vi "pathplan.vi"() -> ()   [LabVIEW 2016]
uses:
  <vilib>/imath/engines/lvmath2/RunTimeEngine/NodeEndStatement/NIMS_NodeEndStatement_Output.vi
  <instcachedir>/0/NIMS_NodeEndStatement_Output_53EC0D466D134D7ABD903AC30B43404B.lvgen/NIMS_NodeEndStatement_Output_53EC0D466D134D7ABD903AC30B43404B_011.vi
  <vilib>/imath/engines/lvmath2/RunTimeEngine/ErrorHandling/NIMS_Finalize Error.vi
panel:
  in  "串口设置（全场定位）":T1={"波特率"=115200, "数据位"=8, "校验"=enum."None", "停止位"=10, "流控制"=0} {"流控制" items=["无"=0, "XON/XOFF"=1, "RTS/CTS"=2, "DTR/DSR"=4]; "停止位" items=["1.0"=10, "1.5"=15, "2.0"=20]; "数据位" min=5 max=8 step=1; "波特率" items=["115200"=115200, "460800"=460800, "75"=75, "110"=110, "134"=134, "150"=150, "300"=300, "600"=600, "1200"=1200, "1800"=1800, "2400"=2400, "4800"=4800, "7200"=7200, "9600"=9600, "14400"=14400, "19200"=19200, "28800"=28800, "38400"=38400, "56000"=56000, "57600"=57600, "128000"=128000, "230400"=230400]}
  in  "全场定位串口":refnum<visa-resource-name>="ASRL4::INSTR" caption="全场定位模块"
  out "起点监视2":sgl[](array[numeric])
  in  "目标位置2":dbl[](array[numeric])=[6000.0, 1500.0]
  out "起点监视3":sgl[](array[numeric])
  in  "目标位置3":dbl[](array[numeric])=[2645.0, 2645.0]
  out "起点监视0":sgl[](array[numeric])
  in  "目标位置0":dbl[](array[numeric])=[12000.0, 0.0]
  in  "Key2(点3)":bool
  in  "Key1(点2)":bool
  in  "Key0(点1)":bool
  in  "speed_max":dbl=15000.0
  in  "发送写入":refnum<visa-resource-name>
  in  "车宽的一半":dbl=200.0
  out "起点监视1":sgl[](array[numeric])
  in  "目标位置1":dbl[](array[numeric])=[9355.0, 2645.0]
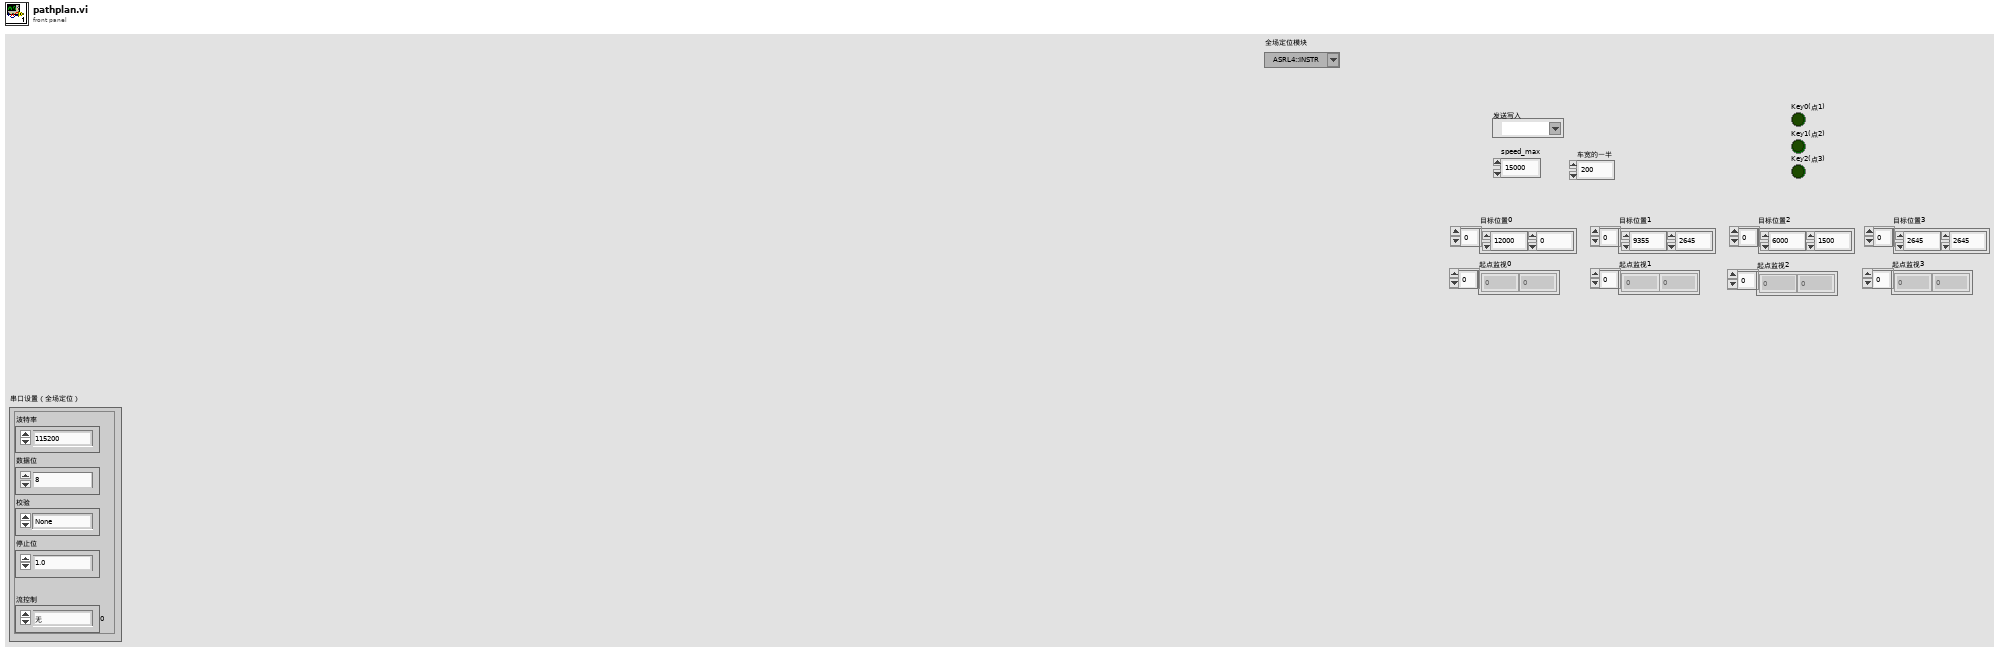
[diagram p1: front panel]
types:
  T1 = cluster{"波特率":u32, "数据位":u16, "校验":enum16{"None", "Odd", "Even", "Mark", "Space"}, "停止位":u16, "流控制":u16}
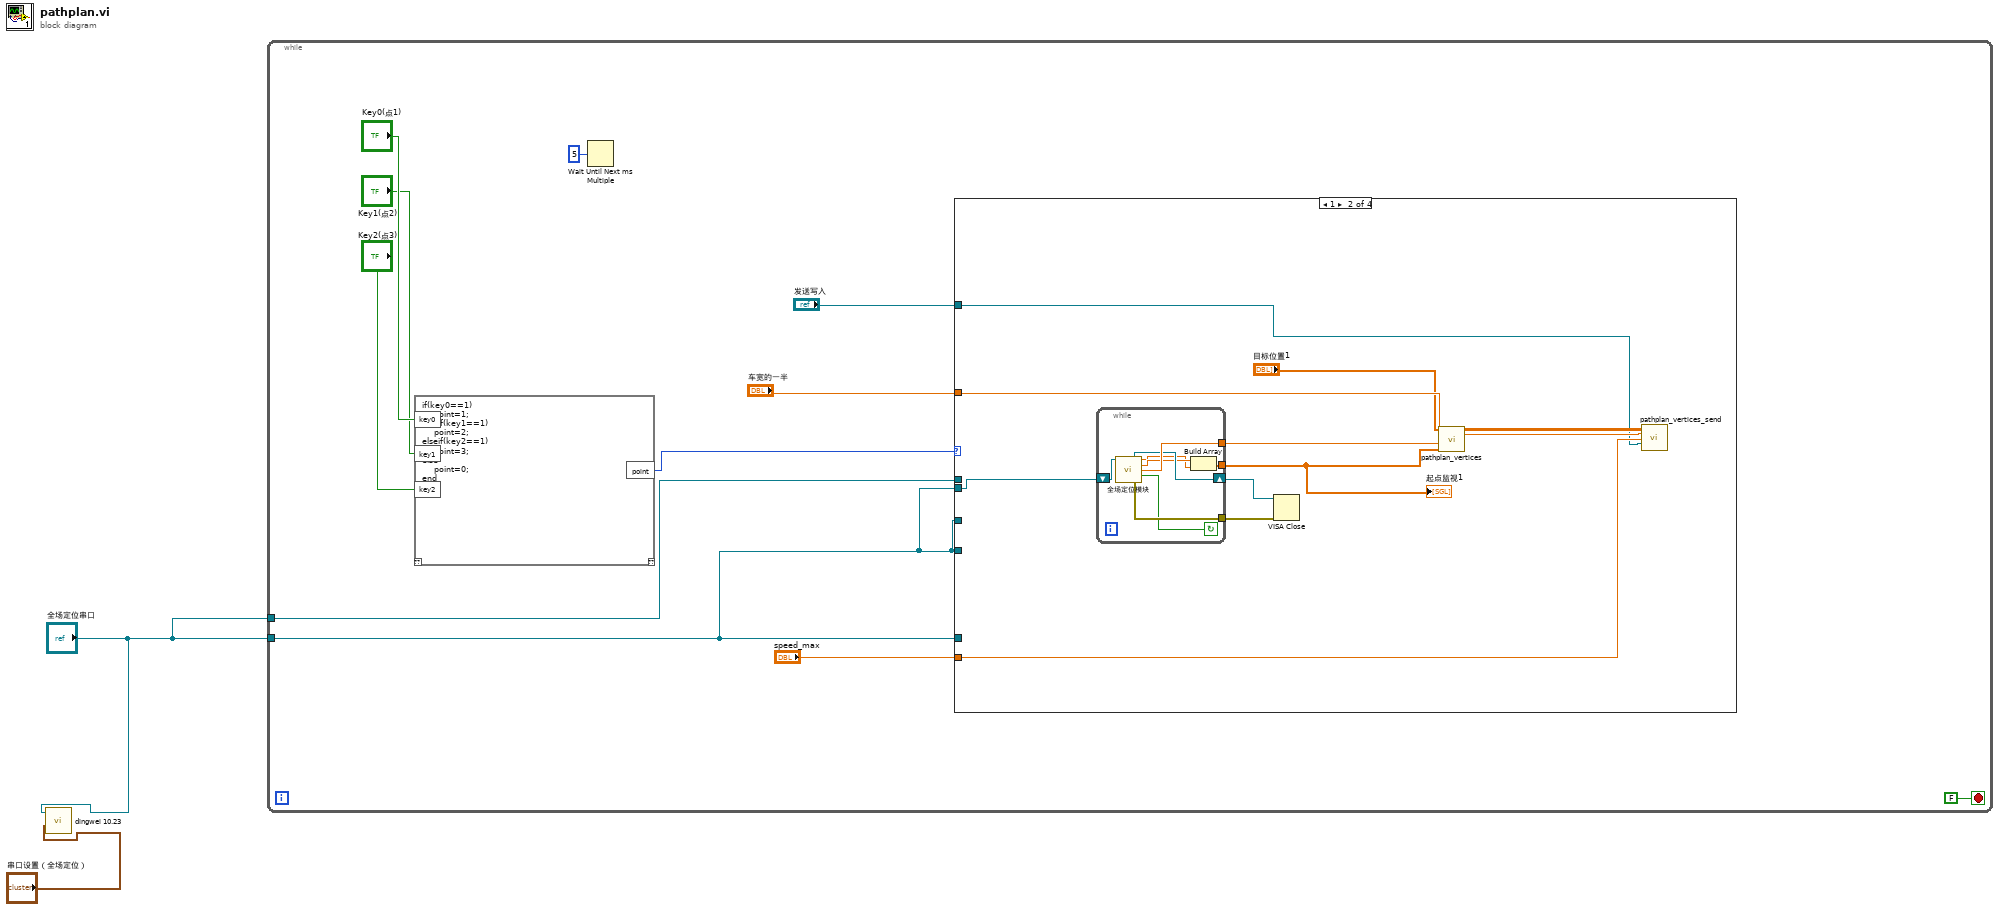
[diagram p0: block diagram]
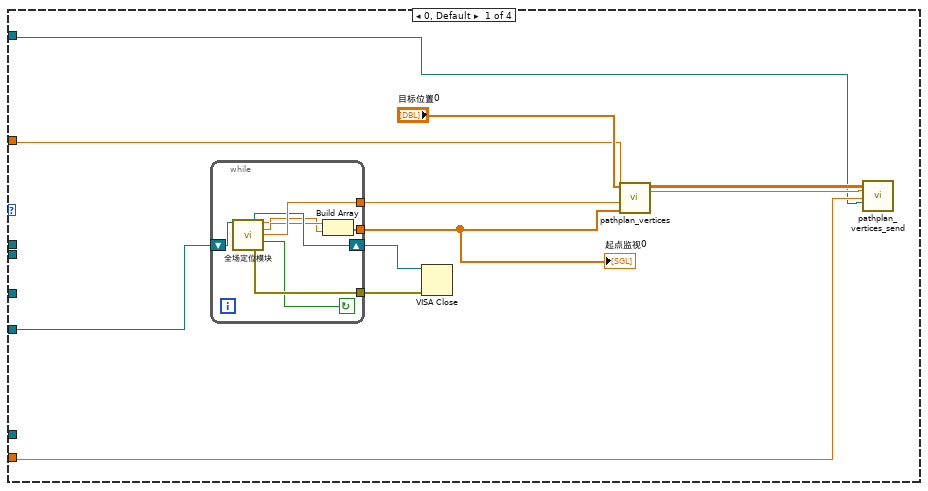
[diagram p2: hidden frame]
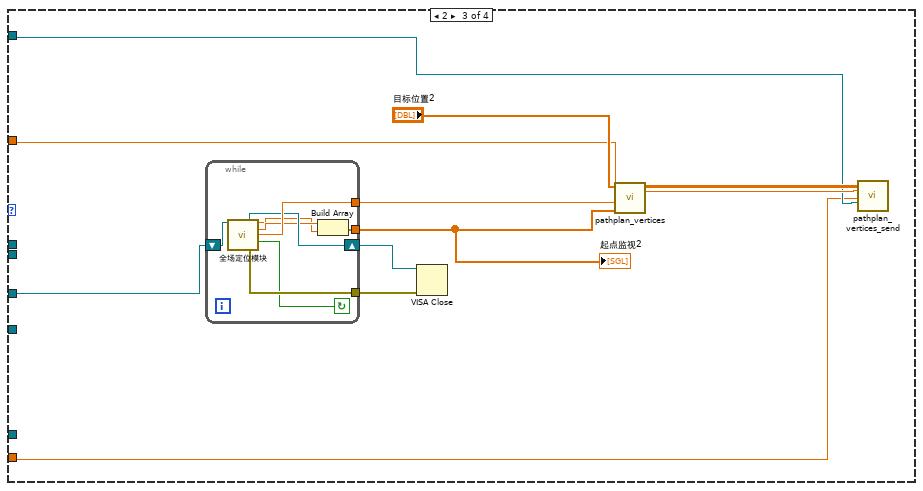
[diagram p3: hidden frame]
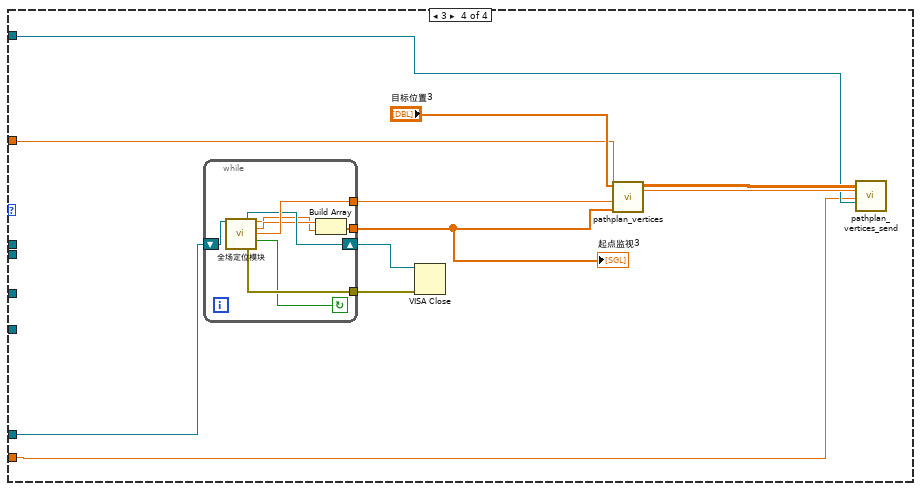
[diagram p4: hidden frame]
diagram:
  n1 = call "dingwei 10.23.vi"("串口设置（遥控器）"="串口设置（全场定位）", "VISA resource name"="全场定位串口") -> ()  [unwired: 10 in]
  n2 = while {
    tunnel: "全场定位串口" -> [w3]
    tunnel: "全场定位串口" -> [w4]
    stop <- FALSE stop-if-true
    n3 = mathscript code="if(key0==1)\n    point=1;\nelseif(key1==1)\n    point=2;\nelseif(key2==1)\n    point=3;\nelse\n    point=0;\nend"("key0"="Key0(点1)", "key1"="Key1(点2)", "key2"="Key2(点3)") -> ("point"=w7:i32)  [unwired: 1 in, 1 out]
    n4 = Wait Until Next ms Multiple(millisecond multiple=u32 5 ("等待时间（毫秒）")) -> ()  [unwired: 1 out]
    n5 = case shown="1" w7 {
      tunnel: "车宽的一半" -> [w92 w118 w130 w149]
      tunnel: "speed_max" -> [w93 w111 w129 w148]
      tunnel: "发送写入" -> [w91 w110 w131 w150]
      tunnel: w3 -> [_ _ _ w147]
      tunnel: w4 -> [_ _ _ _]
      tunnel: w3 -> [w90 _ _ _]
      tunnel: w3 -> [_ _ w128 _]
      tunnel: w3 -> [_ w109 _ _]
      frame 0, Default {
        n6 = while {
          tunnel: [w108] -> w100
          tunnel: [w106] -> w98
          tunnel: [w105] -> w97
          shift-right: [w104] -> w96
          shift-left: w90 -> [w107]
          stop <- w103 continue-if-true
          n7 = call "全场定位模块.vi"("VISA resource name"=w107) -> ("VISA资源名称输出"=w104:refnum<visa-resource-name>, "y"=w101:sgl, "x"=w102:sgl, "Zangle"=w105:sgl, "pd"=w103:bool, "错误输出2"=w106:errorcluster)  [unwired: 8 in, 1 out]
          n8 = Build Array(w102, w101) -> (w108:sgl[])
        }
        "起点监视0" <- w100
        n9 = VISA Close(VISA resource name=w96, error in (no error)=w98) -> ()  [unwired: 1 out]
        n10 = call "pathplan_vertices.vi"("终点"="目标位置0", "车宽的一半"=w92, "z_angle"=w97, "起点"=w100) -> ("vertices"=w95:dbl[][], "distance_all"=w94:dbl)  [unwired: 3 in, 2 out]
        n11 = call "pathplan_vertices_send.vi"("vertices"=w95, "distance_all"=w94, "speed_max"=w93, "写入串口"=w91) -> ()  [unwired: 23 in, 1 out]
      }
      frame 1 {
        n12 = while {
          tunnel: [w127] -> w119
          tunnel: [w125] -> w116
          tunnel: [w124] -> w115
          shift-right: [w123] -> w114
          shift-left: w109 -> [w126]
          stop <- w122 continue-if-true
          n13 = call "全场定位模块.vi"("VISA resource name"=w126) -> ("VISA资源名称输出"=w123:refnum<visa-resource-name>, "y"=w120:sgl, "x"=w121:sgl, "Zangle"=w124:sgl, "pd"=w122:bool, "错误输出2"=w125:errorcluster)  [unwired: 8 in, 1 out]
          n14 = Build Array(w121, w120) -> (w127:sgl[])
        }
        "起点监视1" <- w119
        n15 = VISA Close(VISA resource name=w114, error in (no error)=w116) -> ()  [unwired: 1 out]
        n16 = call "pathplan_vertices.vi"("终点"="目标位置1", "车宽的一半"=w118, "z_angle"=w115, "起点"=w119) -> ("vertices"=w113:dbl[][], "distance_all"=w112:dbl)  [unwired: 3 in, 2 out]
        n17 = call "pathplan_vertices_send.vi"("vertices"=w113, "distance_all"=w112, "speed_max"=w111, "写入串口"=w110) -> ()  [unwired: 23 in, 1 out]
      }
      frame 2 {
        n18 = while {
          tunnel: [w146] -> w138
          tunnel: [w144] -> w136
          tunnel: [w143] -> w135
          shift-right: [w142] -> w134
          shift-left: w128 -> [w145]
          stop <- w141 continue-if-true
          n19 = call "全场定位模块.vi"("VISA resource name"=w145) -> ("VISA资源名称输出"=w142:refnum<visa-resource-name>, "y"=w139:sgl, "x"=w140:sgl, "Zangle"=w143:sgl, "pd"=w141:bool, "错误输出2"=w144:errorcluster)  [unwired: 8 in, 1 out]
          n20 = Build Array(w140, w139) -> (w146:sgl[])
        }
        "起点监视2" <- w138
        n21 = VISA Close(VISA resource name=w134, error in (no error)=w136) -> ()  [unwired: 1 out]
        n22 = call "pathplan_vertices.vi"("终点"="目标位置2", "车宽的一半"=w130, "z_angle"=w135, "起点"=w138) -> ("vertices"=w133:dbl[][], "distance_all"=w132:dbl)  [unwired: 3 in, 2 out]
        n23 = call "pathplan_vertices_send.vi"("vertices"=w133, "distance_all"=w132, "speed_max"=w129, "写入串口"=w131) -> ()  [unwired: 23 in, 1 out]
      }
      frame 3 {
        n24 = while {
          tunnel: [w165] -> w157
          tunnel: [w163] -> w155
          tunnel: [w162] -> w154
          shift-right: [w161] -> w153
          shift-left: w147 -> [w164]
          stop <- w160 continue-if-true
          n25 = call "全场定位模块.vi"("VISA resource name"=w164) -> ("VISA资源名称输出"=w161:refnum<visa-resource-name>, "y"=w158:sgl, "x"=w159:sgl, "Zangle"=w162:sgl, "pd"=w160:bool, "错误输出2"=w163:errorcluster)  [unwired: 8 in, 1 out]
          n26 = Build Array(w159, w158) -> (w165:sgl[])
        }
        "起点监视3" <- w157
        n27 = VISA Close(VISA resource name=w153, error in (no error)=w155) -> ()  [unwired: 1 out]
        n28 = call "pathplan_vertices.vi"("终点"="目标位置3", "车宽的一半"=w149, "z_angle"=w154, "起点"=w157) -> ("vertices"=w152:dbl[][], "distance_all"=w151:dbl)  [unwired: 3 in, 2 out]
        n29 = call "pathplan_vertices_send.vi"("vertices"=w152, "distance_all"=w151, "speed_max"=w148, "写入串口"=w150) -> ()  [unwired: 23 in, 1 out]
      }
    }
  }
